vi "Create Default Attributes.vi"(5 "Unique ID":string, 7 "Process Executive Ref":refnum<data-value>, 11 "Start Low Pressure Wax in":refnum<class "Start Low Pressure Wax.lvclass">) -> (3 "Start Low Pressure Wax out":refnum<class "Start Low Pressure Wax.lvclass">)   [LabVIEW 2019, in "Start Low Pressure Wax.lvclass"]
uses:
  <vilib>/gpm_packages/@cs/Car-wash/Source/Process Steps/Start Low Pressure Wax/Start Low Pressure Wax.lvclass
  <vilib>/gpm_packages/@cs/test-executive/Source/Test Executive/ITestExecutive/ITest Executive.lvclass
  ef3f5f59-afd2-4aa0-8cd3-878208c84f96.vi
  <vilib>/Utility/error.llb/Error Cluster From Error Code.vi
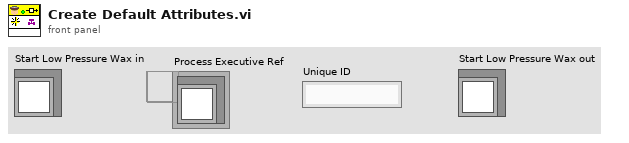
[diagram p1: front panel]
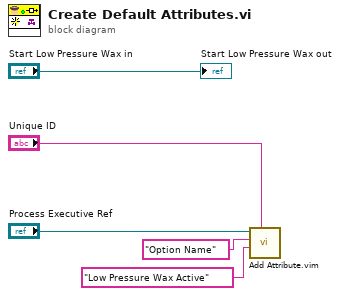
[diagram p0: block diagram]
diagram:
  n1 = call "Add Attribute.vim"("ID"="Unique ID", "Attribute"="Low Pressure Wax Active" ("Item Name"), "Attribute Name"="Option Name" ("Item Name"), "Test Executive Ref"="Process Executive Ref") -> ()  [unwired: 4 in, 4 out]
  "Start Low Pressure Wax out" <- "Start Low Pressure Wax in"
